vi "getrois.vi"(8 "queue in":refnum<queue>, 10 "roi in":T2={[0, 0, 2592, 1944], [{"Contour Type"=0, "ROI Type"=12, [100, 177, 288, 366, 270152]}, {"Contour Type"=0, "ROI Type"=12, [100, 366, 288, 555, 270152]}, {"Contour Type"=0, "ROI Type"=12, [101, 555, 289, 744, 270152]}, {"Contour Type"=0, "ROI Type"=12, [101, 744, 289, 933, 270152]}, {"Contour Type"=0, "ROI Type"=12, [102, 934, 290, 1122, 270152]}, {"Contour Type"=0, "ROI Type"=12, [102, 1123, 290, 1312, 270152]}, {"Contour Type"=0, "ROI Type"=12, [102, 1312, 290, 1501, 270152]}, {"Contour Type"=0, "ROI Type"=12, [103, 1501, 291, 1690, 270152]}, {"Contour Type"=0, "ROI Type"=12, [289, 176, 477, 366, 270152]}, {"Contour Type"=0, "ROI Type"=12, [289, 366, 477, 555, 270152]}, {"Contour Type"=0, "ROI Type"=12, [289, 555, 477, 744, 270152]}, {"Contour Type"=0, "ROI Type"=12, [290, 744, 478, 933, 270152]}, {"Contour Type"=0, "ROI Type"=12, [290, 933, 478, 1122, 270152]}, {"Contour Type"=0, "ROI Type"=12, [290, 1122, 478, 1311, 270152]}, {"Contour Type"=0, "ROI Type"=12, [291, 1311, 479, 1500, 270152]}, {"Contour Type"=0, "ROI Type"=12, [291, 1500, 479, 1689, 270152]}, {"Contour Type"=0, "ROI Type"=12, [477, 176, 665, 365, 270152]}, {"Contour Type"=0, "ROI Type"=12, [478, 365, 666, 554, 270152]}, {"Contour Type"=0, "ROI Type"=12, [478, 554, 666, 743, 270152]}, {"Contour Type"=0, "ROI Type"=12, [478, 743, 666, 932, 270152]}, {"Contour Type"=0, "ROI Type"=12, [479, 932, 667, 1122, 270152]}, {"Contour Type"=0, "ROI Type"=12, [479, 1122, 667, 1311, 270152]}, {"Contour Type"=0, "ROI Type"=12, [479, 1311, 667, 1500, 270152]}, {"Contour Type"=0, "ROI Type"=12, [480, 1500, 668, 1689, 270152]}, {"Contour Type"=0, "ROI Type"=12, [666, 176, 854, 364, 270152]}, {"Contour Type"=0, "ROI Type"=12, [666, 365, 854, 554, 270152]}, {"Contour Type"=0, "ROI Type"=12, [666, 554, 854, 743, 270152]}, {"Contour Type"=0, "ROI Type"=12, [667, 743, 855, 932, 270152]}, {"Contour Type"=0, "ROI Type"=12, [667, 932, 855, 1121, 270152]}, {"Contour Type"=0, "ROI Type"=12, [668, 1121, 856, 1310, 270152]}, {"Contour Type"=0, "ROI Type"=12, [668, 1310, 856, 1499, 270152]}, {"Contour Type"=0, "ROI Type"=12, [668, 1499, 856, 1688, 270152]}, {"Contour Type"=0, "ROI Type"=12, [854, 175, 1042, 364, 270152]}, {"Contour Type"=0, "ROI Type"=12, [855, 364, 1043, 553, 270152]}, {"Contour Type"=0, "ROI Type"=12, [855, 553, 1043, 742, 270152]}, {"Contour Type"=0, "ROI Type"=12, [855, 742, 1043, 931, 270152]}, {"Contour Type"=0, "ROI Type"=12, [856, 932, 1044, 1120, 270152]}, {"Contour Type"=0, "ROI Type"=12, [856, 1121, 1044, 1310, 270152]}, {"Contour Type"=0, "ROI Type"=12, [857, 1310, 1045, 1499, 270152]}, {"Contour Type"=0, "ROI Type"=12, [857, 1499, 1045, 1688, 270152]}, {"Contour Type"=0, "ROI Type"=12, [1043, 174, 1231, 364, 270152]}, {"Contour Type"=0, "ROI Type"=12, [1043, 364, 1231, 553, 270152]}, {"Contour Type"=0, "ROI Type"=12, [1044, 553, 1232, 742, 270152]}, {"Contour Type"=0, "ROI Type"=12, [1044, 742, 1232, 931, 270152]}, {"Contour Type"=0, "ROI Type"=12, [1044, 931, 1232, 1120, 270152]}, {"Contour Type"=0, "ROI Type"=12, [1045, 1120, 1233, 1309, 270152]}, {"Contour Type"=0, "ROI Type"=12, [1045, 1309, 1233, 1498, 270152]}, {"Contour Type"=0, "ROI Type"=12, [1046, 1498, 1234, 1687, 270152]}, {"Contour Type"=0, "ROI Type"=12, [1232, 174, 1420, 363, 270152]}, {"Contour Type"=0, "ROI Type"=12, [1232, 363, 1420, 552, 270152]}, {"Contour Type"=0, "ROI Type"=12, [1232, 552, 1420, 741, 270152]}, {"Contour Type"=0, "ROI Type"=12, [1233, 741, 1421, 930, 270152]}, {"Contour Type"=0, "ROI Type"=12, [1233, 930, 1421, 1120, 270152]}, {"Contour Type"=0, "ROI Type"=12, [1233, 1120, 1421, 1309, 270152]}, {"Contour Type"=0, "ROI Type"=12, [1234, 1309, 1422, 1498, 270152]}, {"Contour Type"=0, "ROI Type"=12, [1234, 1498, 1422, 1687, 270152]}, {"Contour Type"=0, "ROI Type"=12, [1420, 174, 1608, 362, 270152]}, {"Contour Type"=0, "ROI Type"=12, [1420, 363, 1608, 552, 270152]}, {"Contour Type"=0, "ROI Type"=12, [1421, 552, 1609, 741, 270152]}, {"Contour Type"=0, "ROI Type"=12, [1421, 741, 1609, 930, 270152]}, {"Contour Type"=0, "ROI Type"=12, [1422, 930, 1610, 1119, 270152]}, {"Contour Type"=0, "ROI Type"=12, [1422, 1119, 1610, 1308, 270152]}, {"Contour Type"=0, "ROI Type"=12, [1422, 1308, 1610, 1497, 270152]}, {"Contour Type"=0, "ROI Type"=12, [1423, 1497, 1611, 1686, 270152]}, {"Contour Type"=0, "ROI Type"=12, [1609, 173, 1797, 362, 270152]}, {"Contour Type"=0, "ROI Type"=12, [1609, 362, 1797, 551, 270152]}, {"Contour Type"=0, "ROI Type"=12, [1609, 551, 1797, 740, 270152]}, {"Contour Type"=0, "ROI Type"=12, [1610, 740, 1798, 929, 270152]}, {"Contour Type"=0, "ROI Type"=12, [1610, 930, 1798, 1118, 270152]}, {"Contour Type"=0, "ROI Type"=12, [1611, 1119, 1799, 1308, 270152]}, {"Contour Type"=0, "ROI Type"=12, [1611, 1308, 1799, 1497, 270152]}, {"Contour Type"=0, "ROI Type"=12, [1611, 1497, 1799, 1686, 270152]}, {"Contour Type"=0, "ROI Type"=12, [1797, 172, 1985, 362, 270152]}, {"Contour Type"=0, "ROI Type"=12, [1798, 362, 1986, 551, 270152]}, {"Contour Type"=0, "ROI Type"=12, [1798, 551, 1986, 740, 270152]}, {"Contour Type"=0, "ROI Type"=12, [1798, 740, 1986, 929, 270152]}, {"Contour Type"=0, "ROI Type"=12, [1799, 929, 1987, 1118, 270152]}, {"Contour Type"=0, "ROI Type"=12, [1799, 1118, 1987, 1307, 270152]}, {"Contour Type"=0, "ROI Type"=12, [1800, 1307, 1988, 1496, 270152]}, {"Contour Type"=0, "ROI Type"=12, [1800, 1496, 1988, 1685, 270152]}, {"Contour Type"=0, "ROI Type"=12, [1986, 172, 2174, 361, 270152]}, {"Contour Type"=0, "ROI Type"=12, [1986, 361, 2174, 550, 270152]}, {"Contour Type"=0, "ROI Type"=12, [1987, 550, 2175, 739, 270152]}, {"Contour Type"=0, "ROI Type"=12, [1987, 739, 2175, 928, 270152]}, {"Contour Type"=0, "ROI Type"=12, [1987, 928, 2175, 1118, 270152]}, {"Contour Type"=0, "ROI Type"=12, [1988, 1118, 2176, 1307, 270152]}, {"Contour Type"=0, "ROI Type"=12, [1988, 1307, 2176, 1496, 270152]}, {"Contour Type"=0, "ROI Type"=12, [1988, 1496, 2176, 1685, 270152]}, {"Contour Type"=0, "ROI Type"=12, [2174, 172, 2362, 360, 270152]}, {"Contour Type"=0, "ROI Type"=12, [2175, 361, 2363, 550, 270152]}, {"Contour Type"=0, "ROI Type"=12, [2175, 550, 2363, 739, 270152]}, {"Contour Type"=0, "ROI Type"=12, [2176, 739, 2364, 928, 270152]}, {"Contour Type"=0, "ROI Type"=12, [2176, 928, 2364, 1117, 270152]}, {"Contour Type"=0, "ROI Type"=12, [2176, 1117, 2364, 1306, 270152]}, {"Contour Type"=0, "ROI Type"=12, [2177, 1306, 2365, 1495, 270152]}, {"Contour Type"=0, "ROI Type"=12, [2177, 1495, 2365, 1684, 270152]}]}, 11 "image array":i16[][](array[numeric])) -> ()   [LabVIEW 2012]
panel:
  out "Array":T1(array[cluster])
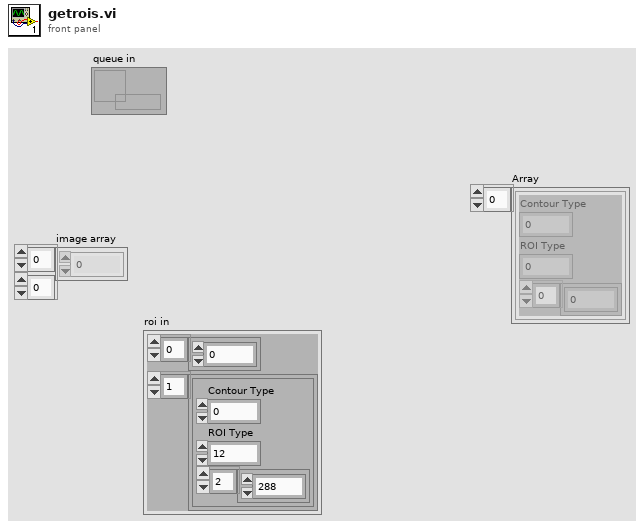
[diagram p1: front panel]
types:
  T1 = cluster{"Contour Type":u32, "ROI Type":u32, i32[]}[]
  T2 = cluster{i32[], cluster{"Contour Type":u32, "ROI Type":u32, i32[]}[]}
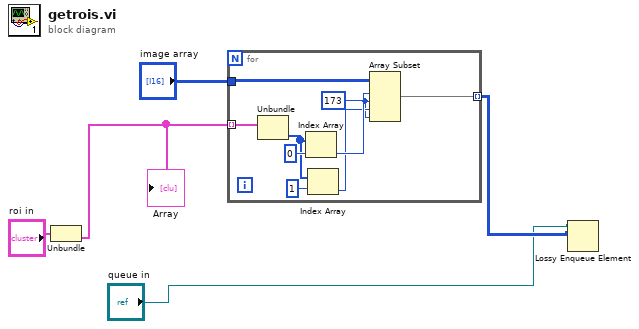
[diagram p0: block diagram]
diagram:
  n1 = Unbundle("roi in") -> (w4:T1)  [unwired: 1 out]
  "Array" <- w4
  n2 = for {
    tunnel: w4 -> [w14] mode=indexing
    tunnel: "image array" -> [w10]
    tunnel: [w6] -> w2 mode=indexing
    w7 = 173 ("length")
    n3 = Unbundle(w14) -> (w12:i32[])  [unwired: 2 out]
    n4 = Index Array(array=w12, index=0) -> (element=w9:i32)
    n5 = Index Array(array=w12, index=1) -> (element=w8:i32)
    n6 = Array Subset(array=w10, index (row)=w9, length (row)=w7, index (col)=w8, length (col)=w7) -> (w6:i16[][])
  }
  n7 = Lossy Enqueue Element(queue="queue in", element=w2) -> ()  [unwired: 1 in, 4 out]
